vi "Next Step.vi"(8 "error in (no error)":errorcluster, 11 "Wavelength PEM and Digikröm in":refnum<class "Wavelength PEM and Digikröm.lvclass">) -> (0 "error out":errorcluster, 1 "Current Step":u32, 2 "Current Position":dbl, 3 "Wavelength PEM and Digikröm out":refnum<class "Wavelength PEM and Digikröm.lvclass">)   [LabVIEW 2017, in "Wavelength PEM and Digikröm.lvclass"]
doc: "(Dynamic) Move to the next preconfigured step of this Scanner, and return the current position (actual, not intended) of this Scanner. Increment the step counter by one."
uses:
  Scanner/Scanner.lvclass
  Instruments/Utility Classes/Scannable/Scannable.lvclass
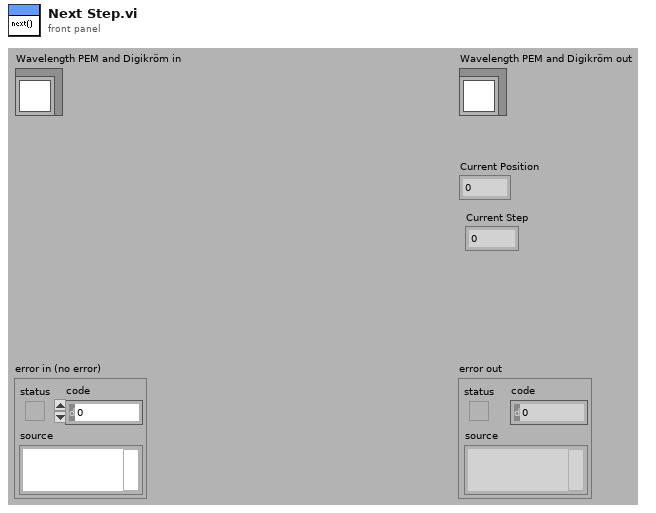
[diagram p1: front panel]
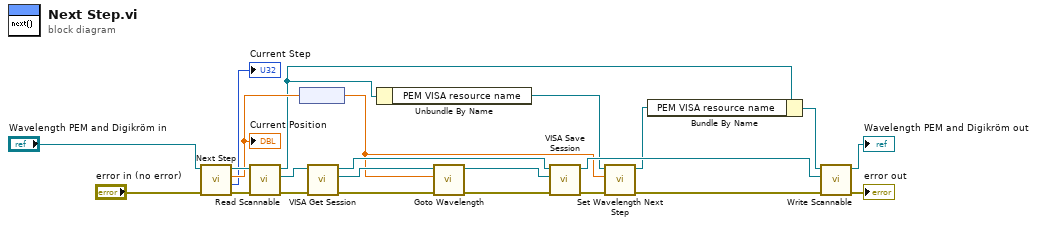
[diagram p0: block diagram]
diagram:
  n1 = call-parent "Next Step.vi"("error in (no error)"="error in (no error)", "Scanner in"="Wavelength PEM and Digikröm in") -> ("error out"=w14:errorcluster, "Current Step"=→"Current Step":u32, "Current Position"=w17:dbl, "Scanner out"=w23:refnum<class "Wavelength PEM and Digikröm.lvclass">)  [unwired: 6 out]
  "Current Position" <- w17
  n2 = call-dynamic "Read Scannable.vi"("error in (no error)"=w14, "Scanner.lvclass in"=w23) -> ("error out"=w13:errorcluster, "Scannable.lvclass"=w18:refnum<class "Scannable.lvclass">, "Scanner.lvclass out"=w5:refnum<class "Wavelength PEM and Digikröm.lvclass">)  [unwired: 7 out]
  n3 = node(w17) -> (w3:dbl[unit])
  n4 = call-dynamic "VISA Get Session.vi"("error in (no error)"=w13, "Instrument.lvclass in"=w18) -> ("error out"=w12:errorcluster, "VISA Resource Name"=w21:refnum<visa-resource-name>, "Instrument.lvclass out"=w22:refnum<class "Scannable.lvclass">)  [unwired: 7 out]
  n5 = Unbundle By Name(w5) -> ("PEM VISA resource name"=w6:refnum<visa-resource-name>)
  n6 = call "Goto Wavelength.vi"("error in (no error)"=w12, "WAVELENGTH"=w3, "VISA resource name"=w21) -> ("error out"=w11:errorcluster, "VISA resource name out"=w20:refnum<visa-resource-name>)  [unwired: 7 out]
  n7 = call-dynamic "VISA Save Session.vi"("error in (no error)"=w11, "VISA Resource Name"=w20, "Instrument.lvclass in"=w22) -> ("error out"=w7:errorcluster, "Instrument.lvclass out"=w19:refnum<class "Scannable.lvclass">)  [unwired: 7 out]
  n8 = call "Set Wavelength Next Step.vi"("error in (no error)"=w7, "wavelength"=w3, "VISA resource name"=w6) -> ("error out"=w2:errorcluster, "VISA resource name out"=w1:refnum<visa-resource-name>)  [unwired: 5 in, 2 out]
  n9 = Bundle By Name(cluster=w5, "PEM VISA resource name"=w1) -> (w4:refnum<class "Wavelength PEM and Digikröm.lvclass">)
  n10 = call-dynamic "Write Scannable.vi"("error in (no error)"=w2, "Scannable.lvclass"=w19, "Scanner.lvclass in"=w4) -> ("error out"=→"error out":errorcluster, "Scanner.lvclass out"=→"Wavelength PEM and Digikröm out":refnum<class "Wavelength PEM and Digikröm.lvclass">)  [unwired: 7 out]
